vi "harp_read_event.vi"(0 "port":refnum<visa-resource-name>, 2 "device ID":u16=1024, 5 "error in (no error)":errorcluster) -> (10 "port":u8, 12 "address":u8 format="%x", 14 "port out":refnum<visa-resource-name>, 15 "payload":T1 {"8 bits" format="%x"}, 16 "n elements":u16, 17 "timestamp":dbl format="%.6f", 19 "error out":errorcluster)   [LabVIEW 2010]
uses:
  <vilib>/Instr/_visa.llb/VISA Configure Serial Port (Instr).vi
panel:
  in  "Boolean":bool
  in  "baud rate":u32(ring)=2000000 items=["250Kbit/s"=250000, "500kbit/s"=500000, "1Mbit/s"=1000000, "2Mbit/s"=2000000, "4Mbit/s"=4000000]
  out "x-y":u32
  out "type":u8(ring)=1 items=["U8"=1, "U16"=2, "U32 "=4, "U64"=8, "I8"=129, "I16"=130, "I32"=132, "I64"=136, "FLOAT"=68, "BOOL"=17]
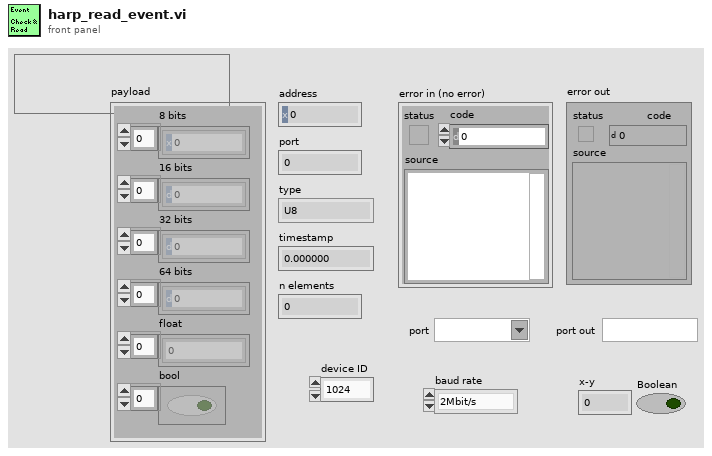
[diagram p1: front panel]
types:
  T1 = cluster{"8 bits":u8[], "bool":bool[], "16 bits":u16[], "32 bits":u32[], "float":sgl[], "64 bits":u64[]}
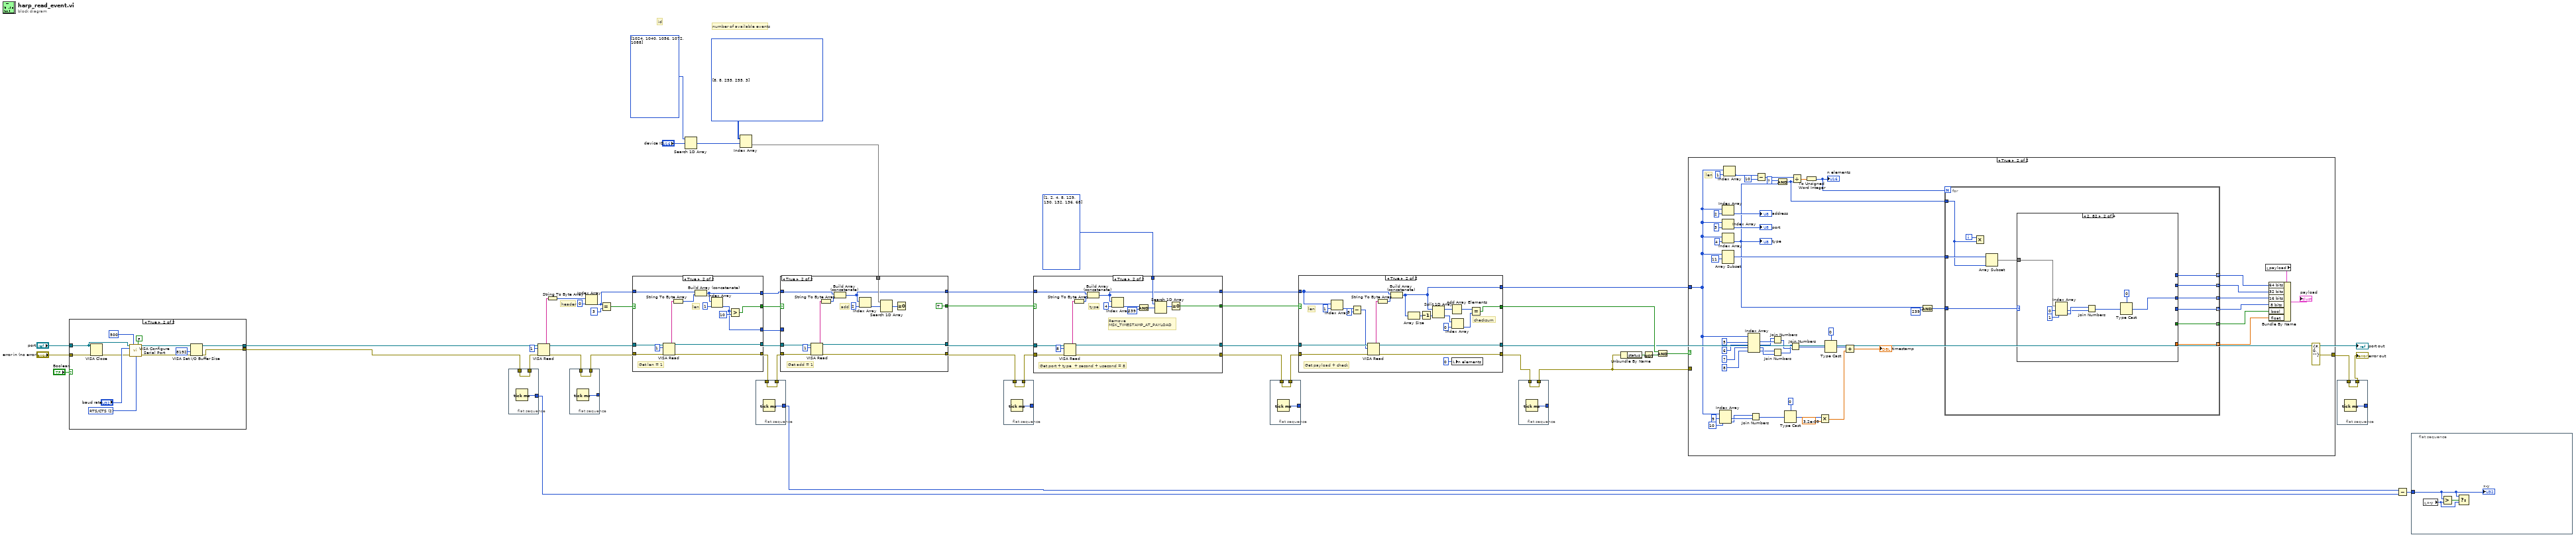
[diagram p0: block diagram]
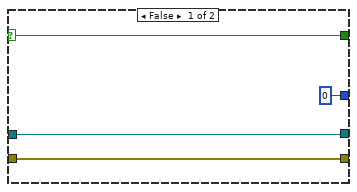
[diagram p6: hidden frame]
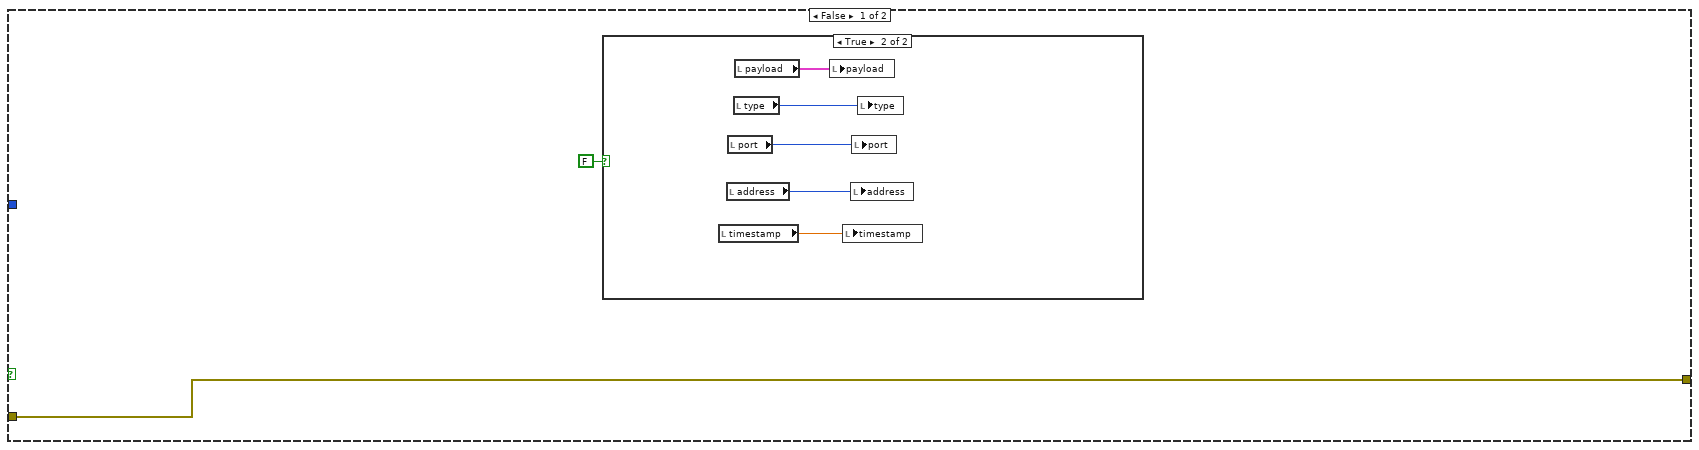
[diagram p7: hidden frame]
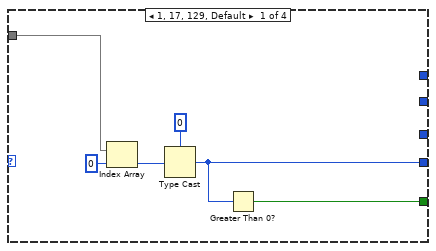
[diagram p9: hidden frame]
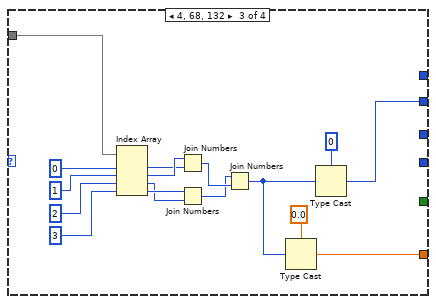
[diagram p10: hidden frame]
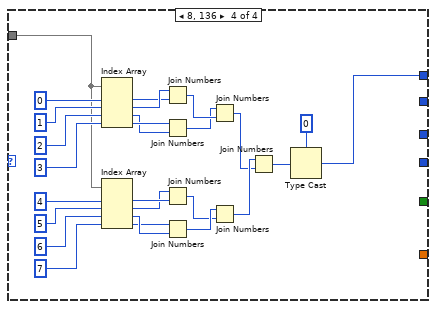
[diagram p11: hidden frame]
diagram:
  w38 = u8[] [1, 2, 4, 8, 129, 130, 132, 136, 68] items=["U8"=1, "U16"=2, "U32 "=4, "U64"=8, "I8"=129, "I16"=130, "I32"=132, "I64"=136, "FLOAT"=68, "BOOL"=17]
  # "header"
  # "number of available events"
  # "id"
  n1 = case shown="True" "Boolean" {
    tunnel: "error in (no error)" -> [w52 w56]
    tunnel: [w52 w58] -> w2
    tunnel: [w53 w57] -> w1
    tunnel: "port" -> [w53 w54]
    frame False {
    }
    frame True {
      w63 = u16 2 items=["None", "XON/XOFF", "RTS/CTS", "XON/XOFF & RTS/CTS", "DTR/DSR", "XON/XOFF & DTR/DSR"] ("flow control (0:none)")
      n2 = VISA Close(VISA resource name=w54, error in (no error)=w56) -> (error out=w55:errorcluster)
      n3 = call-poly "VISA Configure Serial Port"("VISA resource name"=w54, "timeout (10sec)"=u32 500, "Enable Termination\nChar (T)"=FALSE ("Enable Termination\nChar (T)"), "baud rate (9600)"="baud rate", "error in (no error)"=w55, "flow control (0:none)"=w63) -> ("VISA resource name out"=w60:refnum<visa-resource-name>, "error out"=w61:errorcluster)  [unwired: 8 in]
      n4 = VISA Set I/O Buffer Size(VISA resource name=w60, size (4096)=u32 8192, error in (no error)=w61) -> (VISA resource name out=w57:refnum<visa-resource-name>, error out=w58:errorcluster)  [unwired: 1 in]
    }
  }
  n5 = flat-sequence {
    tunnel: w2 -> [w67]
    tunnel: [w67] -> w25
    tunnel: [w66] -> w4
    frame #0 {
      n6 = Tick Count (ms)() -> (millisecond timer value=w66:u32)
    }
  }
  n7 = VISA Read(VISA resource name=w1, byte count=u32 1, error in (no error)=w25) -> (VISA resource name out=w48:refnum<visa-resource-name>, read buffer=w31:string, error out=w24:errorcluster)  [unwired: 1 out]
  n8 = String To Byte Array(string=w31) -> (unsigned byte array=w29:u8[])
  n9 = flat-sequence {
    tunnel: w24 -> [w69]
    tunnel: [w69] -> w23
    tunnel: [w68] -> _
    frame #0 {
      n10 = Tick Count (ms)() -> (millisecond timer value=w68:u32)
    }
  }
  n11 = Index Array(array=w29, index=0) -> (element=w34:u8)
  n12 = Equal?(x=w34, y=u8 3) -> (x = y?=w26:bool)
  n13 = case shown="True" w26 {
    selector: w26 -> [w71 _]
    tunnel: w23 -> [w72 w86]
    tunnel: [w72 w82] -> w22
    tunnel: [w73 w81] -> w45
    tunnel: w48 -> [w73 w79]
    tunnel: w34 -> [_ w77]
    tunnel: [w71 w76] -> w47
    tunnel: [_ w75] -> w46
    tunnel: [u8 0 w74] -> w6
    frame False {
    }
    frame True {
      # "Get len = 1"
      # "len"
      n14 = VISA Read(VISA resource name=w79, byte count=u32 1, error in (no error)=w86) -> (VISA resource name out=w81:refnum<visa-resource-name>, read buffer=w85:string, error out=w82:errorcluster)  [unwired: 1 out]
      n15 = String To Byte Array(string=w85) -> (unsigned byte array=w78:u8[])
      n16 = Build Array (concatenate)(w77, w78) -> (w75:u8[])
      n17 = Index Array(array=w75, index=1) -> (element=w74:u8)
      n18 = Greater?(x=w74, y=u8 10 ("x")) -> (0:w76:bool)
    }
  }
  n19 = Search 1D Array(1D array=u16[] [1024, 1040, 1056, 1072, 1088], element="device ID") -> (index of element=w41:i32)  [unwired: 1 in]
  n20 = Index Array(array=u8[][] [[8], [8], [255], [255], [3]], index (row)=w41) -> (element=w40:u8[])  [unwired: 1 in]
  n21 = flat-sequence {
    tunnel: w22 -> [w88]
    tunnel: [w88] -> w21
    tunnel: [w87] -> w5
    frame #0 {
      n22 = Tick Count (ms)() -> (millisecond timer value=w87:u32)
    }
  }
  n23 = case shown="True" w47 {
    selector: w47 -> [w89 _]
    tunnel: w21 -> [w90 w105]
    tunnel: [w90 w102] -> w13
    tunnel: [w91 w101] -> w12
    tunnel: w45 -> [w91 w100]
    tunnel: w46 -> [_ w98]
    tunnel: w40 -> [_ w97]
    tunnel: [_ w94] -> w39
    tunnel: [w89 TRUE] -> w36
    tunnel: w6 -> [_ _]
    frame False {
    }
    frame True {
      # "Get add = 1"
      # "add"
      n24 = VISA Read(VISA resource name=w100, byte count=u32 1, error in (no error)=w105) -> (VISA resource name out=w101:refnum<visa-resource-name>, read buffer=w104:string, error out=w102:errorcluster)  [unwired: 1 out]
      n25 = String To Byte Array(string=w104) -> (unsigned byte array=w99:u8[])
      n26 = Build Array (concatenate)(w98, w99) -> (w94:u8[])
      n27 = Index Array(array=w94, index=2) -> (element=w96:u8)
      n28 = Search 1D Array(1D array=w97, element=w96) -> (index of element=w95:i32)  [unwired: 1 in]
      n29 = Greater Or Equal To 0?(x=w95) -> ()  [unwired: 1 out]
    }
  }
  n30 = flat-sequence {
    tunnel: w13 -> [w107]
    tunnel: [w107] -> w20
    tunnel: [w106] -> _
    frame #0 {
      n31 = Tick Count (ms)() -> (millisecond timer value=w106:u32)
    }
  }
  n32 = case shown="True" w36 {
    selector: w36 -> [w108 _]
    tunnel: w20 -> [w109 w126]
    tunnel: [w109 w122] -> w11
    tunnel: [w110 w121] -> w10
    tunnel: w12 -> [w110 w120]
    tunnel: w39 -> [_ w118]
    tunnel: w38 -> [_ w117]
    tunnel: [w108 w115] -> w37
    tunnel: [_ w114] -> w35
    frame False {
    }
    frame True {
      # "Remove\nMSK_TIMESTAMP_AT_PAYLOAD"
      # "Get port + type  + second + usecond = 8"
      # "type"
      n33 = VISA Read(VISA resource name=w120, byte count=u32 8, error in (no error)=w126) -> (VISA resource name out=w121:refnum<visa-resource-name>, read buffer=w125:string, error out=w122:errorcluster)  [unwired: 1 out]
      n34 = String To Byte Array(string=w125) -> (unsigned byte array=w119:u8[])
      n35 = Build Array (concatenate)(w118, w119) -> (w114:u8[])
      n36 = Index Array(array=w114, index=4) -> (element=w112:u8)
      n37 = And(x=w112, y=u8 239) -> (x .and. y?=w113:u8)
      n38 = Search 1D Array(1D array=w117, element=w113) -> (index of element=w116:i32)  [unwired: 1 in]
      n39 = Greater Or Equal To 0?(x=w116) -> (x >= 0?=w115:bool)
    }
  }
  n40 = flat-sequence {
    tunnel: w11 -> [w128]
    tunnel: [w128] -> w19
    tunnel: [w127] -> _
    frame #0 {
      n41 = Tick Count (ms)() -> (millisecond timer value=w127:u32)
    }
  }
  n42 = case shown="True" w37 {
    selector: w37 -> [w129 _]
    tunnel: w19 -> [w130 w152]
    tunnel: [w130 w150] -> w18
    tunnel: [w131 w149] -> w3
    tunnel: w10 -> [w131 w148]
    tunnel: w35 -> [_ w143]
    tunnel: [w129 w135] -> w28
    tunnel: [_ w134] -> w27
    frame False {
    }
    frame True {
      # "checksum"
      # "len"
      # "Get payload + check"
      n43 = Index Array(array=w143, index=1) -> (element=w145:u8)
      n44 = Subtract(x=w145, y=u8 9) -> (x-y=w132:u8)
      n45 = VISA Read(VISA resource name=w148, byte count=w132, error in (no error)=w152) -> (VISA resource name out=w149:refnum<visa-resource-name>, read buffer=w151:string, error out=w150:errorcluster)  [unwired: 1 out]
      n46 = String To Byte Array(string=w151) -> (unsigned byte array=w147:u8[])
      n47 = Build Array (concatenate)(w143, w147) -> (w134:u8[])
      n48 = Array Size(array=w134) -> (size(s)=w142:i32)
      n49 = Decrement(x=w142) -> (x-1=w141:i32)
      n50 = Split 1D Array(array=w134, index=w141) -> (first subarray=w140:u8[], second subarray=w137:u8[])
      n51 = Add Array Elements(numeric array=w140) -> (sum=w139:u8)
      n52 = Index Array(array=w137, index=0) -> (element=w136:u8)
      n53 = local write "n elements"(u16 0 ("n elements")) -> ()
      n54 = Equal?(x=w139, y=w136) -> (x = y?=w135:bool)
    }
  }
  "port out" <- w3
  n55 = flat-sequence {
    tunnel: w18 -> [w154]
    tunnel: [w154] -> w17
    tunnel: [w153] -> _
    frame #0 {
      n56 = Tick Count (ms)() -> (millisecond timer value=w153:u32)
    }
  }
  n57 = Unbundle By Name(w17) -> ("status"=w50:bool)
  n58 = Not(x=w50) -> (.not. x?=w49:bool)
  n59 = And(x=w28, y=w49) -> (x .and. y?=w51:bool)
  n60 = case shown="True" w51 {
    tunnel: [w156 errorcluster {"status"=FALSE, "code"=0, "source"=""} ("error out")] -> w16
    tunnel: w27 -> [_ w187]
    tunnel: w17 -> [w156 _]
    frame False {
      n61 = case shown="True" FALSE {
        frame False {
        }
        frame True {
          n62 = local read "timestamp"() -> (w157:dbl)
          n63 = local read "address"() -> (w158:u8)
          n64 = local read "port"() -> (w159:u8)
          n65 = local read "type"() -> (w160:u8)
          n66 = local read "payload"() -> (w161:T1)
          n67 = local write "payload"(w161) -> ()
          n68 = local write "timestamp"(w157) -> ()
          n69 = local write "address"(w158) -> ()
          n70 = local write "port"(w159) -> ()
          n71 = local write "type"(w160) -> ()
        }
      }
    }
    frame True {
      # "len"
      n72 = Index Array(array=w187, index #1=9 ("index"), index #2=10 ("index")) -> (element #1=w181:u8, element #2=w180:u8)
      n73 = Index Array(array=w187, index=2) -> (element=→"address":u8)
      n74 = Index Array(array=w187, index=3) -> (element=→"port":u8)
      n75 = Index Array(array=w187, index=4) -> (element=w185:u8)
      "type" <- w185
      n76 = Array Subset(array=w187, index=11) -> (w200:u8[])  [unwired: 1 in]
      n77 = Index Array(array=w187, index=1) -> (element=w192:u8)
      n78 = Index Array(array=w187, index #1=5 ("index"), index #2=6 ("index"), index #3=7 ("index"), index #4=8 ("index")) -> (element #1=w170:u8, element #2=w166:u8, element #3=w169:u8, element #4=w168:u8)
      n79 = Join Numbers(hi=w180, lo=w181) -> ((hi.lo)=w179:u16)
      n80 = Subtract(x=w192, y=u8 10) -> (x-y=w205:u8)
      n81 = Join Numbers(hi=w166, lo=w170) -> ((hi.lo)=w165:u16)
      n82 = Join Numbers(hi=w168, lo=w169) -> ((hi.lo)=w167:u16)
      n83 = And(x=u8 7, y=w185) -> (x .and. y?=w199:u8)
      n84 = Type Cast(type=u16 0 ("byte count"), x=w179) -> (*(type *) &x=w177:u16)
      n85 = Join Numbers(hi=w167, lo=w165) -> ((hi.lo)=w175:u32)
      n86 = Divide(x=w205, y=w199) -> (x/y=w203:dbl)
      n87 = To Unsigned Word Integer(number=w203) -> (unsigned 16bit integer=w202:u16)
      "n elements" <- w202
      n88 = Multiply(x=w177, y=3.2e-05) -> (x*y=w162:dbl)
      n89 = Type Cast(type=u32 0 ("byte count"), x=w175) -> (*(type *) &x=w163:u32)
      n90 = Add(x=w163, y=w162) -> (x+y=→"timestamp":dbl)
      n91 = And(x=w185, y=u8 239) -> (x .and. y?=w184:u8)
      n92 = for {
        N: w202 -> [_]
        tunnel: w184 -> [w223]
        tunnel: w200 -> [w222]
        tunnel: w199 -> [w220]
        tunnel: [w218] -> w195 mode=indexing
        tunnel: [w217] -> w194 mode=indexing
        tunnel: [w216] -> w198 mode=indexing
        tunnel: [w215] -> w191 mode=indexing
        tunnel: [w214] -> w197 mode=indexing
        tunnel: [w213] -> w196 mode=indexing
        i -> [w221]
        n93 = Multiply(x=w221, y=w220) -> ()  [unwired: 1 out]
        n94 = Array Subset(array=w222, length=w220) -> (w219:u8[])  [unwired: 1 in]
        n95 = case shown="2, 82" w223 {
          tunnel: w219 -> [w226 w231 w240 w255]
          tunnel: [w225 _ _ _] -> w218
          tunnel: [w224 _ _ _] -> w217
          tunnel: [_ w230 _ _] -> w216
          tunnel: [_ _ w239 _] -> w215
          tunnel: [_ _ w238 _] -> w214
          tunnel: [_ _ _ w254] -> w213
          frame 1, 17, 129, Default {
            n96 = Index Array(array=w226, index=0) -> (element=w228:u8)
            n97 = Type Cast(type=u8 0 ("byte count"), x=w228) -> (*(type *) &x=w225:u8)
            n98 = Greater Than 0?(x=w225) -> (x > 0?=w224:bool)
          }
          frame 2, 130 {
            n99 = Index Array(array=w231, index #1=0 ("index"), index #2=1 ("index")) -> (element #1=w234:u8, element #2=w235:u8)
            n100 = Join Numbers(hi=w235, lo=w234) -> ((hi.lo)=w236:u16)
            n101 = Type Cast(type=u16 0 ("byte count"), x=w236) -> (*(type *) &x=w230:u16)
          }
          frame 4, 68, 132 {
            n102 = Index Array(array=w240, index #1=0 ("index"), index #2=1 ("index"), index #3=2 ("index"), index #4=3 ("index")) -> (element #1=w247:u8, element #2=w251:u8, element #3=w248:u8, element #4=w249:u8)
            n103 = Join Numbers(hi=w251, lo=w247) -> ((hi.lo)=w252:u16)
            n104 = Join Numbers(hi=w249, lo=w248) -> ((hi.lo)=w250:u16)
            n105 = Join Numbers(hi=w250, lo=w252) -> ((hi.lo)=w241:u32)
            n106 = Type Cast(type=sgl 0.0 ("byte count"), x=w241) -> (*(type *) &x=w239:sgl)
            n107 = Type Cast(type=u32 0 ("byte count"), x=w241) -> (*(type *) &x=w238:u32)
          }
          frame 8, 136 {
            n108 = Index Array(array=w255, index #1=0 ("index"), index #2=1 ("index"), index #3=2 ("index"), index #4=3 ("index")) -> (element #1=w274:u8, element #2=w278:u8, element #3=w275:u8, element #4=w276:u8)
            n109 = Index Array(array=w255, index #1=4 ("index"), index #2=5 ("index"), index #3=6 ("index"), index #4=7 ("index")) -> (element #1=w265:u8, element #2=w261:u8, element #3=w264:u8, element #4=w263:u8)
            n110 = Join Numbers(hi=w278, lo=w274) -> ((hi.lo)=w279:u16)
            n111 = Join Numbers(hi=w276, lo=w275) -> ((hi.lo)=w277:u16)
            n112 = Join Numbers(hi=w261, lo=w265) -> ((hi.lo)=w260:u16)
            n113 = Join Numbers(hi=w263, lo=w264) -> ((hi.lo)=w262:u16)
            n114 = Join Numbers(hi=w277, lo=w279) -> ((hi.lo)=w258:u32)
            n115 = Join Numbers(hi=w262, lo=w260) -> ((hi.lo)=w259:u32)
            n116 = Join Numbers(hi=w259, lo=w258) -> ((hi.lo)=w256:u64)
            n117 = Type Cast(type=u64 0 ("byte count"), x=w256) -> (*(type *) &x=w254:u64)
          }
        }
      }
      n118 = local read "payload"() -> (w189:T1)
      n119 = Bundle By Name(cluster=w189, "64 bits"=w196, "32 bits"=w197, "16 bits"=w198, "8 bits"=w195, "bool"=w194, "float"=w191) -> (→"payload":T1)
    }
  }
  n120 = flat-sequence {
    tunnel: w16 -> [w281]
    tunnel: [w281] -> w15
    tunnel: [w280] -> _
    frame #0 {
      n121 = Tick Count (ms)() -> (millisecond timer value=w280:u32)
    }
  }
  n122 = Subtract(x=w5, y=w4) -> (x-y=w14:u32)
  n123 = flat-sequence {
    tunnel: w14 -> [w282]
    frame #0 {
      n124 = local read "x-y"() -> (w283:u32)
      n125 = Greater?(x=w282, y=w283) -> (0:w284:bool)
      n126 = Select(t=w282, s=w284, f=w283) -> ()  [unwired: 1 out]
      "x-y" <- w282
    }
  }
  "error out" <- w15
